vi "Measured time.vi"() -> ()   [LabVIEW 2017, in "File.lvlib"]
uses:
  File.lvlib
panel:
  in  "Measured time":timestamp
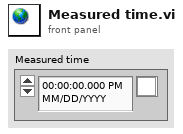
[diagram p1: front panel]
diagram:
